vi "PPMSDR - IV.vi"(10 "Notes":string="fs sweep from 54.8k to 204.8k, 6k step \nT = 590mK\nB=0T\nVbg = -0.55V\nLockin deci: 10\n\nI+/-: 4/2 5mVac +450uVdc, f =0.25\nI2+/-: 28/27 0Vac + 144uVdc\nV+/V-: 27/28\nV2+/V2-: 5/1\nV3+/-: 28/3\n\nfs = 54800", 11 "Experiment folder name":string="20-fs sweep-I-LDr42-RGND-IV") -> ()   [LabVIEW 2013]
uses:
  <vilib>/Analysis/2dsp.llb/Decimate (single shot, DBL).vi
  <userlib>/Levylab/PPMS VI/SubVI/ITX_Global.vi
  <vilib>/Analysis/NI_AALPro.lvlib
panel:
  out "Temp (K)":dbl=0.5907
  out "B Field (Oe)":dbl=-0.061
  out "4Term IV":cluster{dbl[], dbl[]}[](graph)
  out "2Term  IV":cluster{dbl[], dbl[]}[](graph)
  in  "Tab Control":enum32{"Settings", "ITX", "Lockin Data"}(tab)=enum."ITX"
  in  "Gate Channels\n(AO)":i32[](array[numeric])=[2]
  in  "decimating factor":i32=15
  in  "low cutoff freq: fl":dbl=0.01 format="%0.4f"
  in  "offset":dbl[](array[numeric])=[0.0, 0.0, 0.0, 0.0, 0.0, 0.0] format="%_6p"
  in  "invert":dbl[](array[numeric])=[1.0, 1.0, 1.0, 1.0, 1.0, 1.0] format="%#_6p"
  in  "save?":bool=TRUE
  in  "Source AC\nChannels (AO)":i32[](array[numeric])=[0]
  in  "Current Measurement \nChannels (AI)":i32[](array[numeric])=[0, 1]
  in  "Voltage  Measurement\nChannels (AI)":i32[](array[numeric])=[2, 4, 3]
  out "Input signal":waveform(dbl)[](graph)=[{"t0"=timestamp(3559334773.8039565 s since 1904-01-01), "dt"=0.0001824817515283945, "Y"=array[21920 elements], "attributes"=variant("NI_ChannelName"=variant(string "Dev1/ai0"), "NI_UnitDescription"=variant(string "Volts"))}, {"t0"=timestamp(3559334773.8039565 s since 1904-01-01), "dt"=0.0001824817515283945, "Y"=array[21920 elements], "attributes"=variant("NI_ChannelName"=variant(string "Dev1/ai1"), "NI_UnitDescription"=variant(string "Volts"))}, {"t0"=timestamp(3559334773.8039384 s since 1904-01-01), "dt"=0.0001824817515283945, "Y"=array[21920 elements], "attributes"=variant("NI_ChannelName"=variant(string "PXI1Slot8/ai0"), "NI_UnitDescription"=variant(string "Volts"))}, {"t0"=timestamp(3559334773.8039384 s since 1904-01-01), "dt"=0.0001824817515283945, "Y"=array[21920 elements], "attributes"=variant("NI_ChannelName"=variant(string "PXI1Slot8/ai1"), "NI_UnitDescription"=variant(string "Volts"))}, {"t0"=timestamp(3559334773.802993 s since 1904-01-01), "dt"=0.0001824817515283945, "Y"=array[21920 elements], "attributes"=variant("NI_ChannelName"=variant(string "Dev2/ai0"), "NI_UnitDescription"=variant(string "Volts"))}]
  out "output":dbl[][](graph)
  out "time waveform":dbl[](array[numeric])=[3559334774.1414914, 3559334774.1442285, 3559334774.146966, 3559334774.149703, 3559334774.1524405, 3559334774.1551776, 3559334774.1579146, 3559334774.160652, 3559334774.163389, 3559334774.1661263, 3559334774.168864, 3559334774.171601, 3559334774.1743383, 3559334774.1770754, 3559334774.1798124, 3559334774.18255, 3559334774.185287, 3559334774.188024, 3559334774.1907616, 3559334774.1934986, 3559334774.196236, 3559334774.198973, 3559334774.20171, 3559334774.2044477, 3559334774.207185, 3559334774.209922, 3559334774.2126594, 3559334774.2153964, 3559334774.218134, 3559334774.220871, 3559334774.223608, 3559334774.2263455, 3559334774.2290826, 3559334774.23182, 3559334774.234557, 3559334774.237294, 3559334774.2400317, 3559334774.242769, 3559334774.245506, 3559334774.2482433, 3559334774.2509804, 3559334774.253718, 3559334774.256455, 3559334774.259192, 3559334774.2619295, 3559334774.2646666, 3559334774.2674036, 3559334774.270141, 3559334774.272878, 3559334774.2756157, 3559334774.2783527, 3559334774.28109, 3559334774.2838273, 3559334774.2865644, 3559334774.2893014, 3559334774.292039, 3559334774.294776, 3559334774.2975135, 3559334774.3002505, 3559334774.3029876, 3559334774.305725, 3559334774.308462, 3559334774.3111997, 3559334774.3139367, 3559334774.3166738, 3559334774.3194113, 3559334774.3221483, 3559334774.3248854, 3559334774.327623, 3559334774.33036, 3559334774.3330975, 3559334774.3358345, 3559334774.3385715, 3559334774.341309, 3559334774.344046, 3559334774.346783, 3559334774.3495207, 3559334774.3522577, 3559334774.3549953, 3559334774.3577323, 3559334774.3604693, 3559334774.363207, 3559334774.365944, 3559334774.3686814, 3559334774.3714185, 3559334774.3741555, 3559334774.376893, 3559334774.37963, 3559334774.382367, 3559334774.3851047, 3559334774.3878417, 3559334774.390579, 3559334774.3933163, 3559334774.3960533, 3559334774.398791, 3559334774.401528, 3559334774.404265, 3559334774.4070024, 3559334774.4097395, 3559334774.412477, 3559334774.415214, 3559334774.417951, 3559334774.4206886, 3559334774.4234257, 3559334774.4261627, 3559334774.4289002, 3559334774.4316373, 3559334774.434375, 3559334774.437112, 3559334774.439849, 3559334774.4425864, 3559334774.4453235, 3559334774.448061, 3559334774.450798, 3559334774.453535, 3559334774.4562726, 3559334774.4590096, 3559334774.4617467, 3559334774.464484, 3559334774.4672213, 3559334774.469959, 3559334774.472696, 3559334774.475433, 3559334774.4781704, 3559334774.4809074, 3559334774.4836445, 3559334774.486382, 3559334774.489119, 3559334774.4918566, 3559334774.4945936, 3559334774.4973307, 3559334774.500068, 3559334774.502805, 3559334774.5055423, 3559334774.50828, 3559334774.511017, 3559334774.5137544, 3559334774.5164914, 3559334774.5192285, 3559334774.521966, 3559334774.524703, 3559334774.5274405, 3559334774.5301776, 3559334774.5329146, 3559334774.535652, 3559334774.538389, 3559334774.5411263, 3559334774.543864, 3559334774.546601, 3559334774.5493383, 3559334774.5520754, 3559334774.5548124, 3559334774.55755, 3559334774.560287, 3559334774.563024, 3559334774.5657616, 3559334774.5684986, 3559334774.571236, 3559334774.573973, 3559334774.57671, 3559334774.5794477, 3559334774.582185, 3559334774.584922, 3559334774.5876594, 3559334774.5903964, 3559334774.593134, 3559334774.595871, 3559334774.598608, 3559334774.6013455, 3559334774.6040826, 3559334774.60682, 3559334774.609557, 3559334774.612294, 3559334774.6150317, 3559334774.617769, 3559334774.620506, 3559334774.6232433, 3559334774.6259804, 3559334774.628718, 3559334774.631455, 3559334774.634192, 3559334774.6369295, 3559334774.6396666, 3559334774.6424036, 3559334774.645141, 3559334774.647878, 3559334774.6506157, 3559334774.6533527, 3559334774.65609, 3559334774.6588273, 3559334774.6615644, 3559334774.6643014, 3559334774.667039, 3559334774.669776, 3559334774.6725135, 3559334774.6752505, 3559334774.6779876, 3559334774.680725, 3559334774.683462, 3559334774.6861997, 3559334774.6889367, 3559334774.6916738, 3559334774.6944113, 3559334774.6971483, 3559334774.6998854, 3559334774.702623, 3559334774.70536, 3559334774.7080975, 3559334774.7108345, 3559334774.7135715, 3559334774.716309, 3559334774.719046, 3559334774.721783, 3559334774.7245207, 3559334774.7272577, 3559334774.7299953, 3559334774.7327323, 3559334774.7354693, 3559334774.738207, 3559334774.740944, 3559334774.7436814, 3559334774.7464185, 3559334774.7491555, 3559334774.751893, 3559334774.75463, 3559334774.757367, 3559334774.7601047, 3559334774.7628417, 3559334774.765579, 3559334774.7683163, 3559334774.7710533, 3559334774.773791, 3559334774.776528, 3559334774.779265, 3559334774.7820024, 3559334774.7847395, 3559334774.787477, 3559334774.790214, 3559334774.792951, 3559334774.7956886, 3559334774.7984257, 3559334774.8011627, 3559334774.8039002, 3559334774.8066373, 3559334774.809375, 3559334774.812112, 3559334774.814849, 3559334774.8175864, 3559334774.8203235, 3559334774.823061, 3559334774.825798, 3559334774.828535, 3559334774.8312726, 3559334774.8340096, 3559334774.8367467, 3559334774.839484, 3559334774.8422213, 3559334774.844959, 3559334774.847696, 3559334774.850433, 3559334774.8531704, 3559334774.8559074, 3559334774.8586445, 3559334774.861382, 3559334774.864119, 3559334774.8668566, 3559334774.8695936, 3559334774.8723307, 3559334774.875068, 3559334774.877805, 3559334774.8805423, 3559334774.88328, 3559334774.886017, 3559334774.8887544, 3559334774.8914914, 3559334774.8942285, 3559334774.896966, 3559334774.899703, 3559334774.9024405, 3559334774.9051776, 3559334774.9079146, 3559334774.910652, 3559334774.913389, 3559334774.9161263, 3559334774.918864, 3559334774.921601, 3559334774.9243383, 3559334774.9270754, 3559334774.9298124, 3559334774.93255, 3559334774.935287, 3559334774.938024, 3559334774.9407616, 3559334774.9434986, 3559334774.946236, 3559334774.948973, 3559334774.95171, 3559334774.9544477, 3559334774.957185, 3559334774.959922, 3559334774.9626594, 3559334774.9653964, 3559334774.968134, 3559334774.970871, 3559334774.973608, 3559334774.9763455, 3559334774.9790826, 3559334774.98182, 3559334774.984557, 3559334774.987294, 3559334774.9900317, 3559334774.992769, 3559334774.995506, 3559334774.9982433, 3559334775.0009804, 3559334775.003718, 3559334775.006455, 3559334775.009192, 3559334775.0119295, 3559334775.0146666, 3559334775.0174036, 3559334775.020141, 3559334775.022878, 3559334775.0256157, 3559334775.0283527, 3559334775.03109, 3559334775.0338273, 3559334775.0365644, 3559334775.0393014, 3559334775.042039, 3559334775.044776, 3559334775.0475135, 3559334775.0502505, 3559334775.0529876, 3559334775.055725, 3559334775.058462, 3559334775.0611997, 3559334775.0639367, 3559334775.0666738, 3559334775.0694113, 3559334775.0721483, 3559334775.0748854, 3559334775.077623, 3559334775.08036, 3559334775.0830975, 3559334775.0858345, 3559334775.0885715, 3559334775.091309, 3559334775.094046, 3559334775.096783, 3559334775.0995207, 3559334775.1022577, 3559334775.1049953, 3559334775.1077323, 3559334775.1104693, 3559334775.113207, 3559334775.115944, 3559334775.1186814, 3559334775.1214185, 3559334775.1241555, 3559334775.126893, 3559334775.12963, 3559334775.132367, 3559334775.1351047, 3559334775.1378417, 3559334775.140579, 3559334775.1433163, 3559334775.1460533, 3559334775.148791, 3559334775.151528, 3559334775.154265, 3559334775.1570024, 3559334775.1597395, 3559334775.162477, 3559334775.165214, 3559334775.167951, 3559334775.1706886, 3559334775.1734257, 3559334775.1761627, 3559334775.1789002, 3559334775.1816373, 3559334775.184375, 3559334775.187112, 3559334775.189849, 3559334775.1925864, 3559334775.1953235, 3559334775.198061, 3559334775.200798, 3559334775.203535, 3559334775.2062726, 3559334775.2090096, 3559334775.2117467, 3559334775.214484, 3559334775.2172213, 3559334775.219959, 3559334775.222696, 3559334775.225433, 3559334775.2281704, 3559334775.2309074, 3559334775.2336445, 3559334775.236382, 3559334775.239119, 3559334775.2418566, 3559334775.2445936, 3559334775.2473307, 3559334775.250068, 3559334775.252805, 3559334775.2555423, 3559334775.25828, 3559334775.261017, 3559334775.2637544, 3559334775.2664914, 3559334775.2692285, 3559334775.271966, 3559334775.274703, 3559334775.2774405, 3559334775.2801776, 3559334775.2829146, 3559334775.285652, 3559334775.288389, 3559334775.2911263, 3559334775.293864, 3559334775.296601, 3559334775.2993383, 3559334775.3020754, 3559334775.3048124, 3559334775.30755, 3559334775.310287, 3559334775.313024, 3559334775.3157616, 3559334775.3184986, 3559334775.321236, 3559334775.323973, 3559334775.32671, 3559334775.3294477, 3559334775.332185, 3559334775.334922, 3559334775.3376594, 3559334775.3403964, 3559334775.343134, 3559334775.345871, 3559334775.348608, 3559334775.3513455, 3559334775.3540826, 3559334775.35682, 3559334775.359557, 3559334775.362294, 3559334775.3650317, 3559334775.367769, 3559334775.370506, 3559334775.3732433, 3559334775.3759804, 3559334775.378718, 3559334775.381455, 3559334775.384192, 3559334775.3869295, 3559334775.3896666, 3559334775.3924036, 3559334775.395141, 3559334775.397878, 3559334775.4006157, 3559334775.4033527, 3559334775.40609, 3559334775.4088273, 3559334775.4115644, 3559334775.4143014, 3559334775.417039, 3559334775.419776, 3559334775.4225135, 3559334775.4252505, 3559334775.4279876, 3559334775.430725, 3559334775.433462, 3559334775.4361997, 3559334775.4389367, 3559334775.4416738, 3559334775.4444113, 3559334775.4471483, 3559334775.4498854, 3559334775.452623, 3559334775.45536, 3559334775.4580975, 3559334775.4608345, 3559334775.4635715, 3559334775.466309, 3559334775.469046, 3559334775.471783, 3559334775.4745207, 3559334775.4772577, 3559334775.4799953, 3559334775.4827323, 3559334775.4854693, 3559334775.488207, 3559334775.490944, 3559334775.4936814, 3559334775.4964185, 3559334775.4991555, 3559334775.501893, 3559334775.50463, 3559334775.507367, 3559334775.5101047, 3559334775.5128417, 3559334775.515579, 3559334775.5183163, 3559334775.5210533, 3559334775.523791, 3559334775.526528, 3559334775.529265, 3559334775.5320024, 3559334775.5347395, 3559334775.537477, 3559334775.540214, 3559334775.542951, 3559334775.5456886, 3559334775.5484257, 3559334775.5511627, 3559334775.5539002, 3559334775.5566373, 3559334775.559375, 3559334775.562112, 3559334775.564849, 3559334775.5675864, 3559334775.5703235, 3559334775.573061, 3559334775.575798, 3559334775.578535, 3559334775.5812726, 3559334775.5840096, 3559334775.5867467, 3559334775.589484, 3559334775.5922213, 3559334775.594959, 3559334775.597696, 3559334775.600433, 3559334775.6031704, 3559334775.6059074, 3559334775.6086445, 3559334775.611382, 3559334775.614119, 3559334775.6168566, 3559334775.6195936, 3559334775.6223307, 3559334775.625068, 3559334775.627805, 3559334775.6305423, 3559334775.63328, 3559334775.636017, 3559334775.6387544, 3559334775.6414914, 3559334775.6442285, 3559334775.646966, 3559334775.649703, 3559334775.6524405, 3559334775.6551776, 3559334775.6579146, 3559334775.660652, 3559334775.663389, 3559334775.6661263, 3559334775.668864, 3559334775.671601, 3559334775.6743383, 3559334775.6770754, 3559334775.6798124, 3559334775.68255, 3559334775.685287, 3559334775.688024, 3559334775.6907616, 3559334775.6934986, 3559334775.696236, 3559334775.698973, 3559334775.70171, 3559334775.7044477, 3559334775.707185, 3559334775.709922, 3559334775.7126594, 3559334775.7153964, 3559334775.718134, 3559334775.720871, 3559334775.723608, 3559334775.7263455, 3559334775.7290826, 3559334775.73182, 3559334775.734557, 3559334775.737294, 3559334775.7400317, 3559334775.742769, 3559334775.745506, 3559334775.7482433, 3559334775.7509804, 3559334775.753718, 3559334775.756455, 3559334775.759192, 3559334775.7619295, 3559334775.7646666, 3559334775.7674036, 3559334775.770141, 3559334775.772878, 3559334775.7756157, 3559334775.7783527, 3559334775.78109, 3559334775.7838273, 3559334775.7865644, 3559334775.7893014, 3559334775.792039, 3559334775.794776, 3559334775.7975135, 3559334775.8002505, 3559334775.8029876, 3559334775.805725, 3559334775.808462, 3559334775.8111997, 3559334775.8139367, 3559334775.8166738, 3559334775.8194113, 3559334775.8221483, 3559334775.8248854, 3559334775.827623, 3559334775.83036, 3559334775.8330975, 3559334775.8358345, 3559334775.8385715, 3559334775.841309, 3559334775.844046, 3559334775.846783, 3559334775.8495207, 3559334775.8522577, 3559334775.8549953, 3559334775.8577323, 3559334775.8604693, 3559334775.863207, 3559334775.865944, 3559334775.8686814, 3559334775.8714185, 3559334775.8741555, 3559334775.876893, 3559334775.87963, 3559334775.882367, 3559334775.8851047, 3559334775.8878417, 3559334775.890579, 3559334775.8933163, 3559334775.8960533, 3559334775.898791, 3559334775.901528, 3559334775.904265, 3559334775.9070024, 3559334775.9097395, 3559334775.912477, 3559334775.915214, 3559334775.917951, 3559334775.9206886, 3559334775.9234257, 3559334775.9261627, 3559334775.9289002, 3559334775.9316373, 3559334775.934375, 3559334775.937112, 3559334775.939849, 3559334775.9425864, 3559334775.9453235, 3559334775.948061, 3559334775.950798, 3559334775.953535, 3559334775.9562726, 3559334775.9590096, 3559334775.9617467, 3559334775.964484, 3559334775.9672213, 3559334775.969959, 3559334775.972696, 3559334775.975433, 3559334775.9781704, 3559334775.9809074, 3559334775.9836445, 3559334775.986382, 3559334775.989119, 3559334775.9918566, 3559334775.9945936, 3559334775.9973307, 3559334776.000068, 3559334776.002805, 3559334776.0055423, 3559334776.00828, 3559334776.011017, 3559334776.0137544, 3559334776.0164914, 3559334776.0192285, 3559334776.021966, 3559334776.024703, 3559334776.0274405, 3559334776.0301776, 3559334776.0329146, 3559334776.035652, 3559334776.038389, 3559334776.0411263, 3559334776.043864, 3559334776.046601, 3559334776.0493383, 3559334776.0520754, 3559334776.0548124, 3559334776.05755, 3559334776.060287, 3559334776.063024, 3559334776.0657616, 3559334776.0684986, 3559334776.071236, 3559334776.073973, 3559334776.07671, 3559334776.0794477, 3559334776.082185, 3559334776.084922, 3559334776.0876594, 3559334776.0903964, 3559334776.093134, 3559334776.095871, 3559334776.098608, 3559334776.1013455, 3559334776.1040826, 3559334776.10682, 3559334776.109557, 3559334776.112294, 3559334776.1150317, 3559334776.117769, 3559334776.120506, 3559334776.1232433, 3559334776.1259804, 3559334776.128718, 3559334776.131455, 3559334776.134192, 3559334776.1369295, 3559334776.1396666, 3559334776.1424036, 3559334776.145141, 3559334776.147878, 3559334776.1506157, 3559334776.1533527, 3559334776.15609, 3559334776.1588273, 3559334776.1615644, 3559334776.1643014, 3559334776.167039, 3559334776.169776, 3559334776.1725135, 3559334776.1752505, 3559334776.1779876, 3559334776.180725, 3559334776.183462, 3559334776.1861997, 3559334776.1889367, 3559334776.1916738, 3559334776.1944113, 3559334776.1971483, 3559334776.1998854, 3559334776.202623, 3559334776.20536, 3559334776.2080975, 3559334776.2108345, 3559334776.2135715, 3559334776.216309, 3559334776.219046, 3559334776.221783, 3559334776.2245207, 3559334776.2272577, 3559334776.2299953, 3559334776.2327323, 3559334776.2354693, 3559334776.238207, 3559334776.240944, 3559334776.2436814, 3559334776.2464185, 3559334776.2491555, 3559334776.251893, 3559334776.25463, 3559334776.257367, 3559334776.2601047, 3559334776.2628417, 3559334776.265579, 3559334776.2683163, 3559334776.2710533, 3559334776.273791, 3559334776.276528, 3559334776.279265, 3559334776.2820024, 3559334776.2847395, 3559334776.287477, 3559334776.290214, 3559334776.292951, 3559334776.2956886, 3559334776.2984257, 3559334776.3011627, 3559334776.3039002, 3559334776.3066373, 3559334776.309375, 3559334776.312112, 3559334776.314849, 3559334776.3175864, 3559334776.3203235, 3559334776.323061, 3559334776.325798, 3559334776.328535, 3559334776.3312726, 3559334776.3340096, 3559334776.3367467, 3559334776.339484, 3559334776.3422213, 3559334776.344959, 3559334776.347696, 3559334776.350433, 3559334776.3531704, 3559334776.3559074, 3559334776.3586445, 3559334776.361382, 3559334776.364119, 3559334776.3668566, 3559334776.3695936, 3559334776.3723307, 3559334776.375068, 3559334776.377805, 3559334776.3805423, 3559334776.38328, 3559334776.386017, 3559334776.3887544, 3559334776.3914914, 3559334776.3942285, 3559334776.396966, 3559334776.399703, 3559334776.4024405, 3559334776.4051776, 3559334776.4079146, 3559334776.410652, 3559334776.413389, 3559334776.4161263, 3559334776.418864, 3559334776.421601, 3559334776.4243383, 3559334776.4270754, 3559334776.4298124, 3559334776.43255, 3559334776.435287, 3559334776.438024, 3559334776.4407616, 3559334776.4434986, 3559334776.446236, 3559334776.448973, 3559334776.45171, 3559334776.4544477, 3559334776.457185, 3559334776.459922, 3559334776.4626594, 3559334776.4653964, 3559334776.468134, 3559334776.470871, 3559334776.473608, 3559334776.4763455, 3559334776.4790826, 3559334776.48182, 3559334776.484557, 3559334776.487294, 3559334776.4900317, 3559334776.492769, 3559334776.495506, 3559334776.4982433, 3559334776.5009804, 3559334776.503718, 3559334776.506455, 3559334776.509192, 3559334776.5119295, 3559334776.5146666, 3559334776.5174036, 3559334776.520141, 3559334776.522878, 3559334776.5256157, 3559334776.5283527, 3559334776.53109, 3559334776.5338273, 3559334776.5365644, 3559334776.5393014, 3559334776.542039, 3559334776.544776, 3559334776.5475135, 3559334776.5502505, 3559334776.5529876, 3559334776.555725, 3559334776.558462, 3559334776.5611997, 3559334776.5639367, 3559334776.5666738, 3559334776.5694113, 3559334776.5721483, 3559334776.5748854, 3559334776.577623, 3559334776.58036, 3559334776.5830975, 3559334776.5858345, 3559334776.5885715, 3559334776.591309, 3559334776.594046, 3559334776.596783, 3559334776.5995207, 3559334776.6022577, 3559334776.6049953, 3559334776.6077323, 3559334776.6104693, 3559334776.613207, 3559334776.615944, 3559334776.6186814, 3559334776.6214185, 3559334776.6241555, 3559334776.626893, 3559334776.62963, 3559334776.632367, 3559334776.6351047, 3559334776.6378417, 3559334776.640579, 3559334776.6433163, 3559334776.6460533, 3559334776.648791, 3559334776.651528, 3559334776.654265, 3559334776.6570024, 3559334776.6597395, 3559334776.662477, 3559334776.665214, 3559334776.667951, 3559334776.6706886, 3559334776.6734257, 3559334776.6761627, 3559334776.6789002, 3559334776.6816373, 3559334776.684375, 3559334776.687112, 3559334776.689849, 3559334776.6925864, 3559334776.6953235, 3559334776.698061, 3559334776.700798, 3559334776.703535, 3559334776.7062726, 3559334776.7090096, 3559334776.7117467, 3559334776.714484, 3559334776.7172213, 3559334776.719959, 3559334776.722696, 3559334776.725433, 3559334776.7281704, 3559334776.7309074, 3559334776.7336445, 3559334776.736382, 3559334776.739119, 3559334776.7418566, 3559334776.7445936, 3559334776.7473307, 3559334776.750068, 3559334776.752805, 3559334776.7555423, 3559334776.75828, 3559334776.761017, 3559334776.7637544, 3559334776.7664914, 3559334776.7692285, 3559334776.771966, 3559334776.774703, 3559334776.7774405, 3559334776.7801776, 3559334776.7829146, 3559334776.785652, 3559334776.788389, 3559334776.7911263, 3559334776.793864, 3559334776.796601, 3559334776.7993383, 3559334776.8020754, 3559334776.8048124, 3559334776.80755, 3559334776.810287, 3559334776.813024, 3559334776.8157616, 3559334776.8184986, 3559334776.821236, 3559334776.823973, 3559334776.82671, 3559334776.8294477, 3559334776.832185, 3559334776.834922, 3559334776.8376594, 3559334776.8403964, 3559334776.843134, 3559334776.845871, 3559334776.848608, 3559334776.8513455, 3559334776.8540826, 3559334776.85682, 3559334776.859557, 3559334776.862294, 3559334776.8650317, 3559334776.867769, 3559334776.870506, 3559334776.8732433, 3559334776.8759804, 3559334776.878718, 3559334776.881455, 3559334776.884192, 3559334776.8869295, 3559334776.8896666, 3559334776.8924036, 3559334776.895141, 3559334776.897878, 3559334776.9006157, 3559334776.9033527, 3559334776.90609, 3559334776.9088273, 3559334776.9115644, 3559334776.9143014, 3559334776.917039, 3559334776.919776, 3559334776.9225135, 3559334776.9252505, 3559334776.9279876, 3559334776.930725, 3559334776.933462, 3559334776.9361997, 3559334776.9389367, 3559334776.9416738, 3559334776.9444113, 3559334776.9471483, 3559334776.9498854, 3559334776.952623, 3559334776.95536, 3559334776.9580975, 3559334776.9608345, 3559334776.9635715, 3559334776.966309, 3559334776.969046, 3559334776.971783, 3559334776.9745207, 3559334776.9772577, 3559334776.9799953, 3559334776.9827323, 3559334776.9854693, 3559334776.988207, 3559334776.990944, 3559334776.9936814, 3559334776.9964185, 3559334776.9991555, 3559334777.001893, 3559334777.00463, 3559334777.007367, 3559334777.0101047, 3559334777.0128417, 3559334777.015579, 3559334777.0183163, 3559334777.0210533, 3559334777.023791, 3559334777.026528, 3559334777.029265, 3559334777.0320024, 3559334777.0347395, 3559334777.037477, 3559334777.040214, 3559334777.042951, 3559334777.0456886, 3559334777.0484257, 3559334777.0511627, 3559334777.0539002, 3559334777.0566373, 3559334777.059375, 3559334777.062112, 3559334777.064849, 3559334777.0675864, 3559334777.0703235, 3559334777.073061, 3559334777.075798, 3559334777.078535, 3559334777.0812726, 3559334777.0840096, 3559334777.0867467, 3559334777.089484, 3559334777.0922213, 3559334777.094959, 3559334777.097696, 3559334777.100433, 3559334777.1031704, 3559334777.1059074, 3559334777.1086445, 3559334777.111382, 3559334777.114119, 3559334777.1168566, 3559334777.1195936, 3559334777.1223307, 3559334777.125068, 3559334777.127805, 3559334777.1305423, 3559334777.13328, 3559334777.136017, 3559334777.1387544, 3559334777.1414914, 3559334777.1442285, 3559334777.146966, 3559334777.149703, 3559334777.1524405, 3559334777.1551776, 3559334777.1579146, 3559334777.160652, 3559334777.163389, 3559334777.1661263, 3559334777.168864, 3559334777.171601, 3559334777.1743383, 3559334777.1770754, 3559334777.1798124, 3559334777.18255, 3559334777.185287, 3559334777.188024, 3559334777.1907616, 3559334777.1934986, 3559334777.196236, 3559334777.198973, 3559334777.20171, 3559334777.2044477, 3559334777.207185, 3559334777.209922, 3559334777.2126594, 3559334777.2153964, 3559334777.218134, 3559334777.220871, 3559334777.223608, 3559334777.2263455, 3559334777.2290826, 3559334777.23182, 3559334777.234557, 3559334777.237294, 3559334777.2400317, 3559334777.242769, 3559334777.245506, 3559334777.2482433, 3559334777.2509804, 3559334777.253718, 3559334777.256455, 3559334777.259192, 3559334777.2619295, 3559334777.2646666, 3559334777.2674036, 3559334777.270141, 3559334777.272878, 3559334777.2756157, 3559334777.2783527, 3559334777.28109, 3559334777.2838273, 3559334777.2865644, 3559334777.2893014, 3559334777.292039, 3559334777.294776, 3559334777.2975135, 3559334777.3002505, 3559334777.3029876, 3559334777.305725, 3559334777.308462, 3559334777.3111997, 3559334777.3139367, 3559334777.3166738, 3559334777.3194113, 3559334777.3221483, 3559334777.3248854, 3559334777.327623, 3559334777.33036, 3559334777.3330975, 3559334777.3358345, 3559334777.3385715, 3559334777.341309, 3559334777.344046, 3559334777.346783, 3559334777.3495207, 3559334777.3522577, 3559334777.3549953, 3559334777.3577323, 3559334777.3604693, 3559334777.363207, 3559334777.365944, 3559334777.3686814, 3559334777.3714185, 3559334777.3741555, 3559334777.376893, 3559334777.37963, 3559334777.382367, 3559334777.3851047, 3559334777.3878417, 3559334777.390579, 3559334777.3933163, 3559334777.3960533, 3559334777.398791, 3559334777.401528, 3559334777.404265, 3559334777.4070024, 3559334777.4097395, 3559334777.412477, 3559334777.415214, 3559334777.417951, 3559334777.4206886, 3559334777.4234257, 3559334777.4261627, 3559334777.4289002, 3559334777.4316373, 3559334777.434375, 3559334777.437112, 3559334777.439849, 3559334777.4425864, 3559334777.4453235, 3559334777.448061, 3559334777.450798, 3559334777.453535, 3559334777.4562726, 3559334777.4590096, 3559334777.4617467, 3559334777.464484, 3559334777.4672213, 3559334777.469959, 3559334777.472696, 3559334777.475433, 3559334777.4781704, 3559334777.4809074, 3559334777.4836445, 3559334777.486382, 3559334777.489119, 3559334777.4918566, 3559334777.4945936, 3559334777.4973307, 3559334777.500068, 3559334777.502805, 3559334777.5055423, 3559334777.50828, 3559334777.511017, 3559334777.5137544, 3559334777.5164914, 3559334777.5192285, 3559334777.521966, 3559334777.524703, 3559334777.5274405, 3559334777.5301776, 3559334777.5329146, 3559334777.535652, 3559334777.538389, 3559334777.5411263, 3559334777.543864, 3559334777.546601, 3559334777.5493383, 3559334777.5520754, 3559334777.5548124, 3559334777.55755, 3559334777.560287, 3559334777.563024, 3559334777.5657616, 3559334777.5684986, 3559334777.571236, 3559334777.573973, 3559334777.57671, 3559334777.5794477, 3559334777.582185, 3559334777.584922, 3559334777.5876594, 3559334777.5903964, 3559334777.593134, 3559334777.595871, 3559334777.598608, 3559334777.6013455, 3559334777.6040826, 3559334777.60682, 3559334777.609557, 3559334777.612294, 3559334777.6150317, 3559334777.617769, 3559334777.620506, 3559334777.6232433, 3559334777.6259804, 3559334777.628718, 3559334777.631455, 3559334777.634192, 3559334777.6369295, 3559334777.6396666, 3559334777.6424036, 3559334777.645141, 3559334777.647878, 3559334777.6506157, 3559334777.6533527, 3559334777.65609, 3559334777.6588273, 3559334777.6615644, 3559334777.6643014, 3559334777.667039, 3559334777.669776, 3559334777.6725135, 3559334777.6752505, 3559334777.6779876, 3559334777.680725, 3559334777.683462, 3559334777.6861997, 3559334777.6889367, 3559334777.6916738, 3559334777.6944113, 3559334777.6971483, 3559334777.6998854, 3559334777.702623, 3559334777.70536, 3559334777.7080975, 3559334777.7108345, 3559334777.7135715, 3559334777.716309, 3559334777.719046, 3559334777.721783, 3559334777.7245207, 3559334777.7272577, 3559334777.7299953, 3559334777.7327323, 3559334777.7354693, 3559334777.738207, 3559334777.740944, 3559334777.7436814, 3559334777.7464185, 3559334777.7491555, 3559334777.751893, 3559334777.75463, 3559334777.757367, 3559334777.7601047, 3559334777.7628417, 3559334777.765579, 3559334777.7683163, 3559334777.7710533, 3559334777.773791, 3559334777.776528, 3559334777.779265, 3559334777.7820024, 3559334777.7847395, 3559334777.787477, 3559334777.790214, 3559334777.792951, 3559334777.7956886, 3559334777.7984257, 3559334777.8011627, 3559334777.8039002, 3559334777.8066373, 3559334777.809375, 3559334777.812112, 3559334777.814849, 3559334777.8175864, 3559334777.8203235, 3559334777.823061, 3559334777.825798, 3559334777.828535, 3559334777.8312726, 3559334777.8340096, 3559334777.8367467, 3559334777.839484, 3559334777.8422213, 3559334777.844959, 3559334777.847696, 3559334777.850433, 3559334777.8531704, 3559334777.8559074, 3559334777.8586445, 3559334777.861382, 3559334777.864119, 3559334777.8668566, 3559334777.8695936, 3559334777.8723307, 3559334777.875068, 3559334777.877805, 3559334777.8805423, 3559334777.88328, 3559334777.886017, 3559334777.8887544, 3559334777.8914914, 3559334777.8942285, 3559334777.896966, 3559334777.899703, 3559334777.9024405, 3559334777.9051776, 3559334777.9079146, 3559334777.910652, 3559334777.913389, 3559334777.9161263, 3559334777.918864, 3559334777.921601, 3559334777.9243383, 3559334777.9270754, 3559334777.9298124, 3559334777.93255, 3559334777.935287, 3559334777.938024, 3559334777.9407616, 3559334777.9434986, 3559334777.946236, 3559334777.948973, 3559334777.95171, 3559334777.9544477, 3559334777.957185, 3559334777.959922, 3559334777.9626594, 3559334777.9653964, 3559334777.968134, 3559334777.970871, 3559334777.973608, 3559334777.9763455, 3559334777.9790826, 3559334777.98182, 3559334777.984557, 3559334777.987294, 3559334777.9900317, 3559334777.992769, 3559334777.995506, 3559334777.9982433, 3559334778.0009804, 3559334778.003718, 3559334778.006455, 3559334778.009192, 3559334778.0119295, 3559334778.0146666, 3559334778.0174036, 3559334778.020141, 3559334778.022878, 3559334778.0256157, 3559334778.0283527, 3559334778.03109, 3559334778.0338273, 3559334778.0365644, 3559334778.0393014, 3559334778.042039, 3559334778.044776, 3559334778.0475135, 3559334778.0502505, 3559334778.0529876, 3559334778.055725, 3559334778.058462, 3559334778.0611997, 3559334778.0639367, 3559334778.0666738, 3559334778.0694113, 3559334778.0721483, 3559334778.0748854, 3559334778.077623, 3559334778.08036, 3559334778.0830975, 3559334778.0858345, 3559334778.0885715, 3559334778.091309, 3559334778.094046, 3559334778.096783, 3559334778.0995207, 3559334778.1022577, 3559334778.1049953, 3559334778.1077323, 3559334778.1104693, 3559334778.113207, 3559334778.115944, 3559334778.1186814, 3559334778.1214185, 3559334778.1241555, 3559334778.126893, 3559334778.12963, 3559334778.132367, 3559334778.1351047, 3559334778.1378417]
  out "All DC Voltages":dbl[](array[numeric])=[0.00045, 0.000144, 0.0, 0.0]
  out "current time":timestamp=timestamp(3559334775.883591 s since 1904-01-01)
  # "IV Config Channel Settings"
  # "Filter/Data  Settings"
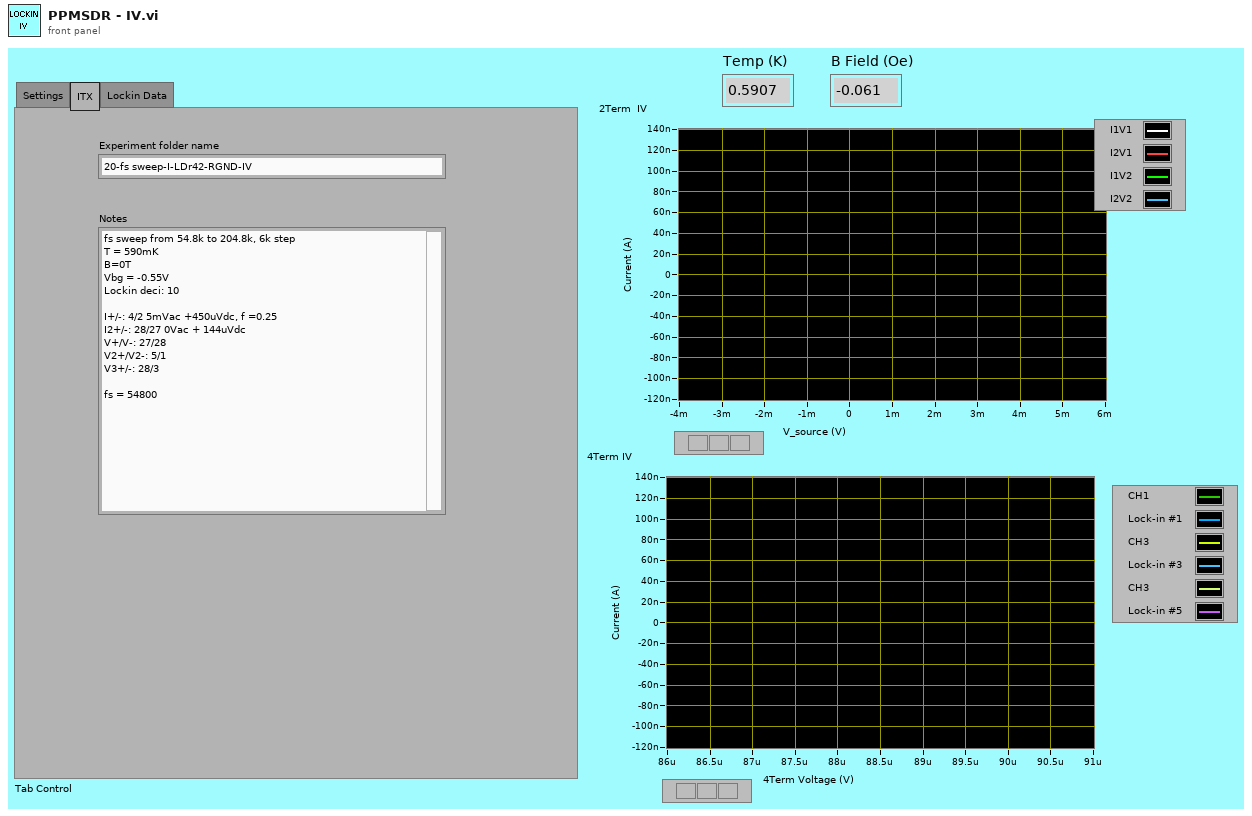
[diagram p1: front panel]
types:
  T1 = cluster{"AO amp (V)":dbl[], "AO DC (V)":dbl[], "AO f (Hz)":dbl[], "AO phi (deg)":dbl[], "function":enum16{"Sine Wave", "Triangle Wave", "Square Wave", "Sawtooth Wave"}[]}
  T2 = cluster{"Decimated Array":dbl[], "Decimated Array":dbl[]}
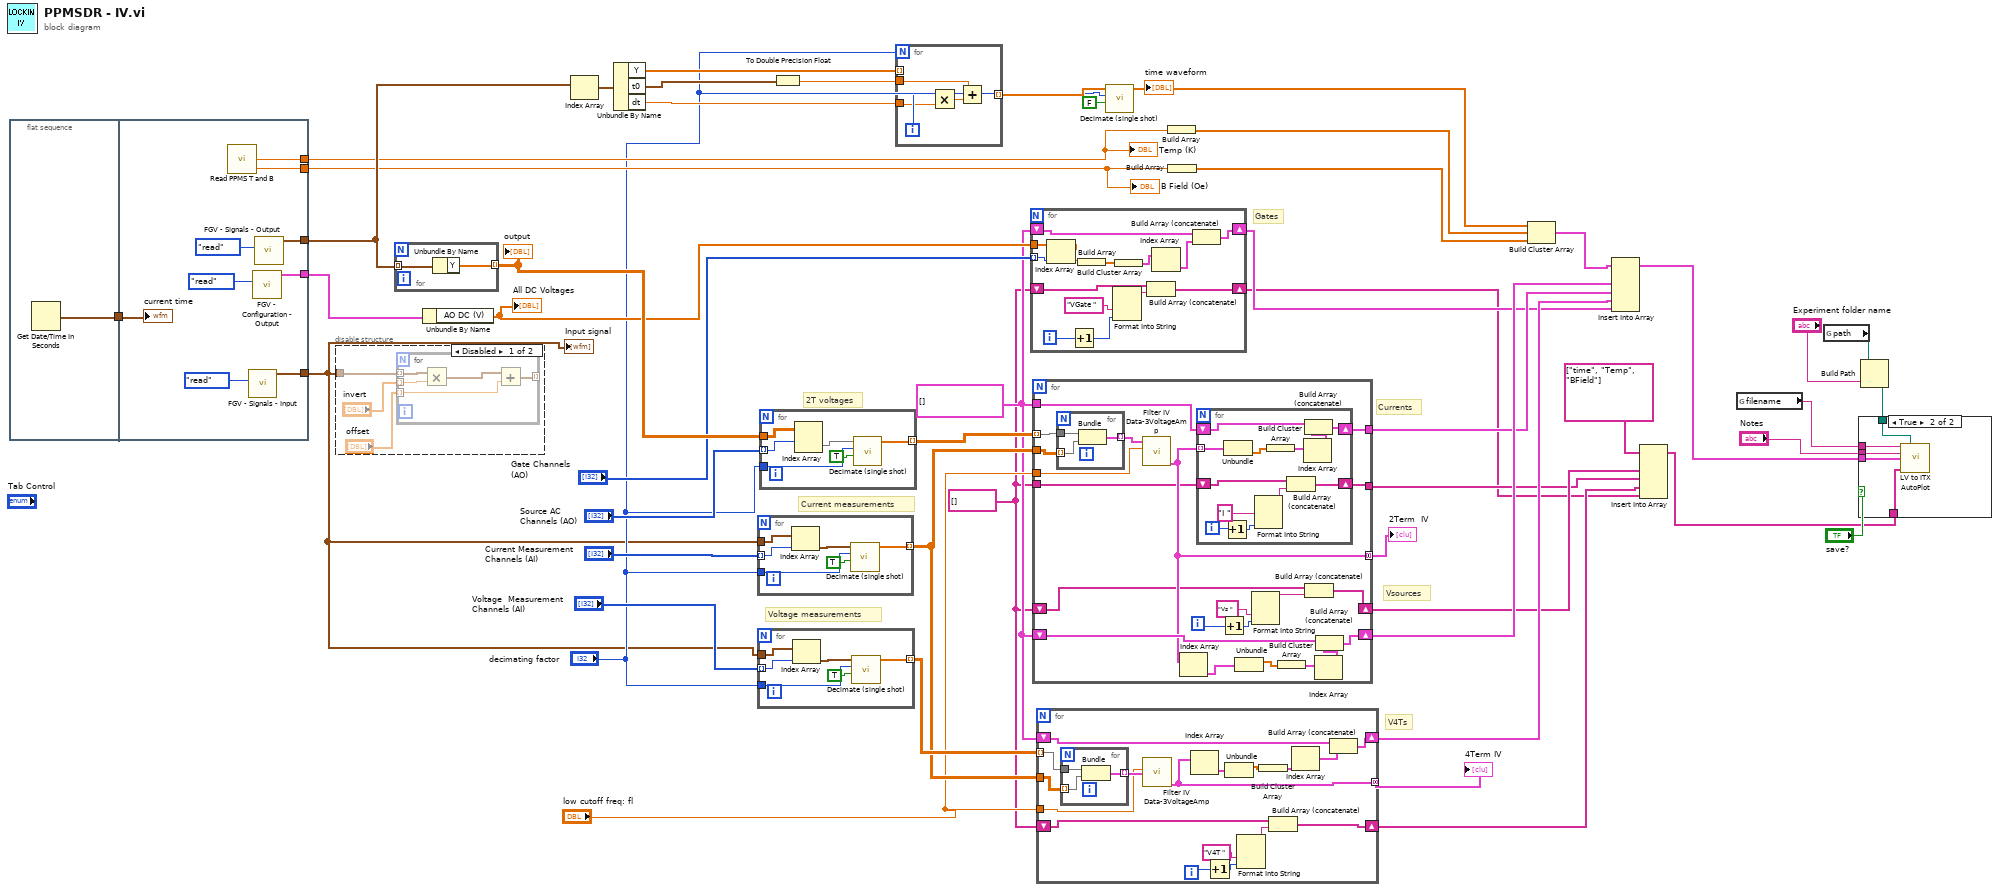
[diagram p0: block diagram]
diagram:
  w22 = string[] []
  w23 = cluster{dbl[]}[] []
  # "V4Ts"
  # "Vsources"
  # "Currents"
  # "Gates"
  # "Voltage measurements"
  # "Current measurements"
  # "2T voltages"
  n1 = flat-sequence {
    tunnel: [w50] -> w1
    tunnel: [w55] -> w2
    tunnel: [w58] -> w39
    tunnel: [w52] -> w4
    tunnel: [w56] -> w26
    tunnel: w1 -> [w53]
    tunnel: [w51] -> w5
    frame #0 {
      n2 = Get Date/Time In Seconds() -> (seconds since 1Jan1904=w50:timestamp)
    }
    frame #1 {
      n3 = call <userlib>:"Read PPMS T and B.vi"() -> ("Field"=w52:dbl, "Temperature"=w51:dbl)  [unwired: 3 in, 1 out]
      n4 = call <userlib>:"FGV - Signals - Input.vi"("Function"=enum16{"write", "read"}."read") -> ("input signal"=w55:waveform(dbl)[])  [unwired: 5 in, 1 out]
      n5 = call <userlib>:"FGV - Configuration - Output.vi"("Function"=enum16{"write", "read"}."read") -> ("Channels: AO 2"=w56:T1)  [unwired: 5 in, 1 out]
      n6 = call <userlib>:"FGV - Signals - Output.vi"("Function"=enum16{"write", "read"}."read") -> ("input signal"=w58:waveform(dbl)[])  [unwired: 5 in, 1 out]
      "current time" <- w53
    }
  }
  n7 = disable-structure shown="Disabled" {
    disable-tunnel: w2 -> [w60 _]
    frame Disabled {
      n8 = for {
        tunnel: w60 -> [w66] mode=indexing
        tunnel: [w67] -> _ mode=indexing
        tunnel: "offset" -> [w64] mode=indexing
        tunnel: "invert" -> [w65] mode=indexing
        n9 = Multiply(x=w66, y=w65) -> (x*y=w63:waveform(dbl))
        n10 = Add(x=w63, y=w64) -> (x+y=w67:waveform(dbl))
      }
    }
    frame Enabled {
    }
  }
  n11 = for {
    tunnel: w39 -> [w69] mode=indexing
    tunnel: [w68] -> w27 mode=indexing
    n12 = Unbundle By Name(w69) -> ("Y"=w68:dbl[])
  }
  "output" <- w27
  n13 = Unbundle By Name(w26) -> ("AO DC (V)"=w25:dbl[])
  "All DC Voltages" <- w25
  n14 = Index Array(array=w39) -> (element=w38:waveform(dbl))  [unwired: 1 in]
  n15 = Unbundle By Name(w38) -> ("Y"=w37:dbl[], "t0"=w40:timestamp, "dt"=w41:dbl)
  n16 = for {
    tunnel: "Current Measurement \nChannels (AI)" -> [w75] mode=indexing
    tunnel: w2 -> [w74]
    tunnel: "decimating factor" -> [w71]
    tunnel: [w70] -> w30 mode=indexing
    n17 = Index Array(array=w74, index=w75) -> (element=w72:waveform(dbl))
    n18 = call-poly <vilib>:"Decimate (single shot).vi"("averaging"=TRUE, "decimating factor"=w71, "X"=w72) -> ("Decimated Array"=w70:dbl[])  [unwired: 7 in, 1 out]
  }
  n19 = for {
    tunnel: "Voltage  Measurement\nChannels (AI)" -> [w81] mode=indexing
    tunnel: w2 -> [w80]
    tunnel: "decimating factor" -> [w77]
    tunnel: [w76] -> w31 mode=indexing
    n20 = Index Array(array=w80, index=w81) -> (element=w78:waveform(dbl))
    n21 = call-poly <vilib>:"Decimate (single shot).vi"("averaging"=TRUE, "decimating factor"=w77, "X"=w78) -> ("Decimated Array"=w76:dbl[])  [unwired: 7 in, 1 out]
  }
  n22 = for {
    tunnel: "Source AC\nChannels (AO)" -> [w87] mode=indexing
    tunnel: w27 -> [w86]
    tunnel: "decimating factor" -> [w83]
    tunnel: [w82] -> w34 mode=indexing
    n23 = Index Array(array=w86, index (row)=w87) -> (element=w84:dbl[])  [unwired: 1 in]
    n24 = call-poly <vilib>:"Decimate (single shot).vi"("averaging"=TRUE, "decimating factor"=w83, "X"=w84) -> ("Decimated Array"=w82:dbl[])  [unwired: 7 in, 1 out]
  }
  n25 = To Double Precision Float(number=w40) -> (double precision float=w43:dbl)
  n26 = for {
    N: "decimating factor" -> [_]
    tunnel: w41 -> [w91]
    tunnel: w43 -> [w89]
    tunnel: [w88] -> w42 mode=indexing
    tunnel: w37 -> [_] mode=indexing
    i -> [w92]
    n27 = Multiply(x=w92, y=w91) -> (x*y=w90:dbl)
    n28 = Add(x=w89, y=w90) -> (x+y=w88:dbl)
  }
  n29 = for {
    tunnel: w25 -> [w106]
    tunnel: "Gate Channels\n(AO)" -> [w105] mode=indexing
    shift-right: [w97] -> w14
    shift-left: w23 -> [w96]
    shift-right: [w94] -> w9
    shift-left: w22 -> [w93]
    i -> [w95]
    n30 = Index Array(array=w106, index=w105) -> (element=w99:dbl)
    n31 = Increment(x=w95) -> (x+1=w100:i32)
    n32 = Build Array(w99) -> (w98:dbl[])
    n33 = Format Into String("VGate ", w100) -> (resulting string=w102:string)  [unwired: 3 in, 1 out]
    n34 = Build Cluster Array(w98) -> (w104:cluster{dbl[]}[])
    n35 = Build Array (concatenate)(w93, w102) -> (w94:string[])
    n36 = Index Array(array=w104) -> (element=w103:cluster{dbl[]})  [unwired: 1 in]
    n37 = Build Array (concatenate)(w96, w103) -> (w97:cluster{dbl[]}[])
  }
  n38 = for {
    tunnel: w34 -> [w127] mode=indexing
    tunnel: w30 -> [w126]
    tunnel: "low cutoff freq: fl" -> [w124]
    tunnel: [w117] -> w33 mode=concatenating
    tunnel: [w123] -> w16
    shift-right: [w120] -> w17
    shift-left: w23 -> [w118]
    tunnel: w23 -> [w119]
    tunnel: [w114] -> w11
    tunnel: w22 -> [w113]
    shift-right: [w110] -> w12
    shift-left: w22 -> [w111]
    i -> [w107]
    n39 = for {
      tunnel: w127 -> [w142]
      tunnel: w126 -> [w141] mode=indexing
      tunnel: [w140] -> w125 mode=indexing
      n40 = Bundle("Decimated Array"=w142, "Decimated Array"=w141) -> (w140:T2)  [unwired: 1 in]
    }
    n41 = call <userlib>:"Filter IV Data-3VoltageAmp.vi"("low cutoff freq: fl"=w124, "Four terminal IVs"=w125) -> ("V vs I 2"=w117:cluster{dbl[], dbl[]}[])  [unwired: 1 in]
    n42 = Index Array(array=w117) -> (element=w116:cluster{dbl[], dbl[]})  [unwired: 1 in]
    n43 = for {
      shift-right: [w139] -> w123
      shift-left: w119 -> [w138]
      tunnel: w117 -> [w137] mode=indexing
      shift-right: [w129] -> w114
      shift-left: w113 -> [w128]
      i -> [w132]
      n44 = Increment(x=w132) -> (x+1=w131:i32)
      n45 = Unbundle(w137) -> (w136:dbl[])  [unwired: 1 out]
      n46 = Format Into String("I ", w131) -> (resulting string=w130:string)  [unwired: 3 in, 1 out]
      n47 = Build Cluster Array(w136) -> (w135:cluster{dbl[]}[])
      n48 = Build Array (concatenate)(w128, w130) -> (w129:string[])
      n49 = Index Array(array=w135) -> (element=w134:cluster{dbl[]})  [unwired: 1 in]
      n50 = Build Array (concatenate)(w138, w134) -> (w139:cluster{dbl[]}[])
    }
    n51 = Increment(x=w107) -> (x+1=w108:i32)
    n52 = Unbundle(w116) -> (w115:dbl[])  [unwired: 1 out]
    n53 = Format Into String("Vs ", w108) -> (resulting string=w112:string)  [unwired: 3 in, 1 out]
    n54 = Build Cluster Array(w115) -> (w122:cluster{dbl[]}[])
    n55 = Build Array (concatenate)(w111, w112) -> (w110:string[])
    n56 = Index Array(array=w122) -> (element=w121:cluster{dbl[]})  [unwired: 1 in]
    n57 = Build Array (concatenate)(w118, w121) -> (w120:cluster{dbl[]}[])
  }
  "2Term  IV" <- w33
  n58 = for {
    tunnel: w31 -> [w159] mode=indexing
    tunnel: w30 -> [w158]
    tunnel: "low cutoff freq: fl" -> [w156]
    tunnel: [w146] -> w28 mode=concatenating
    shift-right: [w148] -> w10
    shift-left: w22 -> [w147]
    shift-right: [w144] -> w15
    shift-left: w23 -> [w143]
    i -> [w145]
    n59 = for {
      tunnel: w159 -> [w162]
      tunnel: w158 -> [w161] mode=indexing
      tunnel: [w160] -> w157 mode=indexing
      n60 = Bundle("Decimated Array"=w162, "Decimated Array"=w161) -> (w160:T2)  [unwired: 1 in]
    }
    n61 = call <userlib>:"Filter IV Data-3VoltageAmp.vi"("low cutoff freq: fl"=w156, "Four terminal IVs"=w157) -> ("V vs I 2"=w146:cluster{dbl[], dbl[]}[])  [unwired: 1 in]
    n62 = Index Array(array=w146) -> (element=w153:cluster{dbl[], dbl[]})  [unwired: 1 in]
    n63 = Increment(x=w145) -> (x+1=w149:i32)
    n64 = Unbundle(w153) -> (w152:dbl[])  [unwired: 1 out]
    n65 = Format Into String("V4T ", w149) -> (resulting string=w151:string)  [unwired: 3 in, 1 out]
    n66 = Build Cluster Array(w152) -> (w155:cluster{dbl[]}[])
    n67 = Build Array (concatenate)(w147, w151) -> (w148:string[])
    n68 = Index Array(array=w155) -> (element=w154:cluster{dbl[]})  [unwired: 1 in]
    n69 = Build Array (concatenate)(w143, w154) -> (w144:cluster{dbl[]}[])
  }
  "4Term IV" <- w28
  n70 = call-poly <vilib>:"Decimate (single shot).vi"("averaging"=FALSE, "decimating factor"="decimating factor", "X"=w42) -> ("Decimated Array"=w21:dbl[])  [unwired: 7 in, 1 out]
  "time waveform" <- w21
  n71 = Build Array(w5) -> (w20:dbl[])
  n72 = Build Array(w4) -> (w19:dbl[])
  n73 = Build Cluster Array(w21, w20, w19) -> (w18:cluster{"Decimated Array":dbl[]}[])
  n74 = Insert Into Array(array=w18, new element #1=w17, new element #2=w16, new element #3=w15, new element #4=w14) -> (w6:cluster{"Decimated Array":dbl[]}[])  [unwired: 1 in]
  n75 = Insert Into Array(array=string[] ["time", "Temp", "BField"] ("wavenames (.Vx, etc)"), new element #1=w12, new element #2=w11, new element #3=w10, new element #4=w9) -> (w7:string[])  [unwired: 1 in]
  n76 = global read "ITX_Global.vi" "filename"() -> (w45:string)
  n77 = global read "ITX_Global.vi" "path"() -> (w48:path)
  n78 = Build Path(base path=w48, name or relative path="Experiment folder name") -> (appended path=w46:path)
  n79 = case shown="True" "save?" {
    tunnel: w46 -> [_ w167]
    tunnel: "Notes" -> [_ w166]
    tunnel: w45 -> [_ w165]
    tunnel: w7 -> [_ w164]
    tunnel: w6 -> [_ w163]
    frame False {
    }
    frame True {
      n80 = call <userlib>:"LV to ITX AutoPlot.vi"("filename"=w165, "path"=w167, "Notes"=w166, "Data"=w163, "wavenames (.Vx, etc)"=w164) -> ()  [unwired: 10 in, 1 out]
    }
  }
  "Input signal" <- w2
  "Temp (K)" <- w5
  "B Field (Oe)" <- w4
